vi "servoTest.vi"() -> ()   [LabVIEW 2018]
uses:
  <vilib>/LabVIEW Interface for Arduino/LabVIEW Interface for Arduino.lvlib
panel:
  in  "VISA resource":refnum<visa-resource-name>="COM11"
  in  "Servo 1 Angle Input 2":u8(knob) scale=35.0..75.0
  in  "Servo 2 Angle Input":u8(knob) scale=120.0..160.0
  in  "Stop":bool
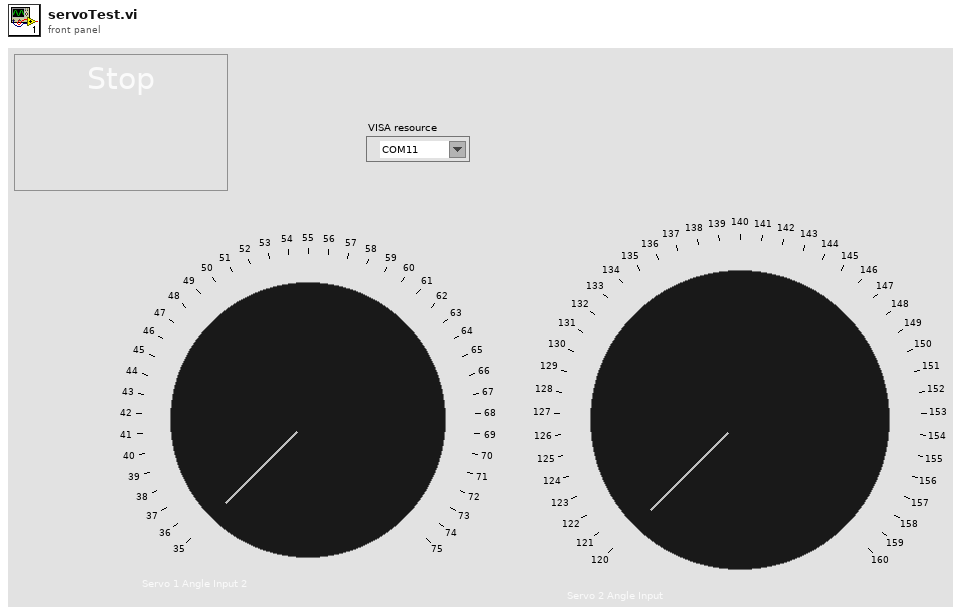
[diagram p1: front panel]
types:
  T1 = typedef "LabVIEW Interface for Arduino.lvlib/Arduino Resource.ctl" = cluster{"VISA resource":refnum<visa-resource-name>, "Board Type":T2, "Connection Type":enum8{"USB / Serial"}, "Bytes Per Packet (15)":u8}
  T2 = typedef "LabVIEW Interface for Arduino.lvlib/Board Type.ctl" = enum16{"Uno", "Dimuelanove w/Atmega 328", "Mega 2560"}
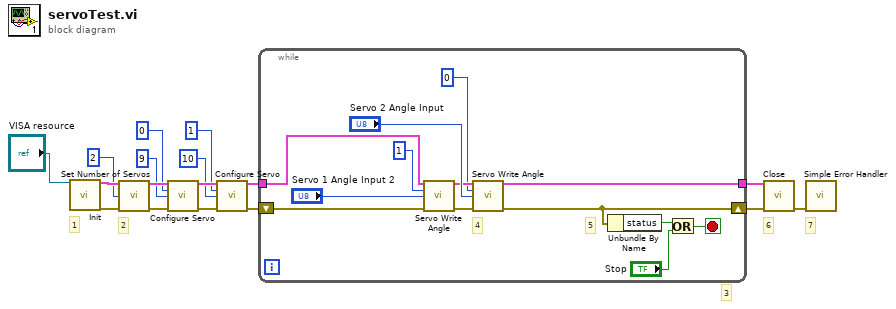
[diagram p0: block diagram]
diagram:
  # "7"
  # "6"
  # "3"
  # "2"
  # "1"
  n1 = call <vilib>:"Init.vi"("VISA resource"="VISA resource") -> ("Arduino Resource"=w17:T1, "error out"=w16:errorcluster)  [unwired: 17 in]
  n2 = call <vilib>:"Set Number of Servos.vi"("Arduino Resource"=w17, "Number Of Servos (1)"=u8 2 ("Number of Servos"), "error in"=w16) -> ("Arduino Resource"=w14:T1, "error out"=w13:errorcluster)  [unwired: 11 in]
  n3 = call <vilib>:"Configure Servo.vi"("Arduino Resource"=w14, "Servo Number (0)"=u8 0 ("Servo Number"), "DIO Pin (2)"=u8 9 ("Servo Number"), "error in"=w13) -> ("Arduino Resource"=w12:T1, "error out"=w11:errorcluster)  [unwired: 10 in]
  n4 = call <vilib>:"Configure Servo.vi"("Arduino Resource"=w12, "Servo Number (0)"=u8 1 ("Servo Number"), "DIO Pin (2)"=u8 10 ("Servo Number"), "error in"=w11) -> ("Arduino Resource"=w6:T1, "error out"=w5:errorcluster)  [unwired: 10 in]
  n5 = while {
    tunnel: w6 -> [w30]
    tunnel: [w20] -> w3
    shift-right: [w19] -> w4
    shift-left: w5 -> [w29]
    stop <- w27 stop-if-true
    # "5"
    # "4"
    n6 = call <vilib>:"Servo Write Angle.vi"("Arduino Resource"=w30, "Servo Number"=u8 1, "Angle (Degrees)"="Servo 1 Angle Input 2", "error in"=w29) -> ("Arduino Resource"=w23:T1, "error out"=w22:errorcluster)  [unwired: 10 in]
    n7 = call <vilib>:"Servo Write Angle.vi"("Arduino Resource"=w23, "Servo Number"=u8 0, "Angle (Degrees)"="Servo 2 Angle Input", "error in"=w22) -> ("Arduino Resource"=w20:T1, "error out"=w19:errorcluster)  [unwired: 10 in]
    n8 = Unbundle By Name(w19) -> ("status"=w26:bool)
    n9 = Or(x=w26, y="Stop") -> (x .or. y?=w27:bool)
  }
  n10 = call <vilib>:"Close.vi"("Arduino Resource"=w3, "error in"=w4) -> ("error out"=w1:errorcluster)  [unwired: 13 in]
  n11 = call <vilib>:"Simple Error Handler.vi"("error in (no error)"=w1) -> ()  [unwired: 4 in, 5 out]
